vi "getSetup.vi"(7 "Monochromator in":T1={"Type"=enum."PTI", "Wavelength (nm)"=0.0, "Grating, gr/mm"=enum."2400", "Grating mode"=enum."Unknown", "Spectrum mode"={"Spectrum mode?"=FALSE, "Start wavelength (nm)"=0.0, "End wavelength (nm)"=0.0, "Wavelength step (nm)"=0.0, "Wavelength array"=[], "array index"=0}, "PTI"={"Delay before read (ms)"=0, "Mono 1"={"Timeout (ms)"=0, "Resource Name"="", "Baud Rate"=0, "Data Bits"=0, "Parity"=0, "Stop Bits"=0, "Flow Control"=0}, "Mono 2"={"Timeout (ms)"=0, "Resource Name"="", "Baud Rate"=0, "Data Bits"=0, "Parity"=0, "Stop Bits"=0, "Flow Control"=0}, "Two PTI Monochromators?"=FALSE}, "Oriel (custom)"={"reference"=refnum}, "Force wavelength confirmation (PTI)?"=FALSE} {"PTI"."Mono 2"."Flow Control" items=["1.0"=10, "1.5"=15, "2.0"=20]; "PTI"."Mono 2"."Stop Bits" items=["None", "Odd", "Even", "Mark", "Space"]; "PTI"."Mono 2"."Parity" items=["None", "Odd", "Even", "Mark", "Space"]; "PTI"."Mono 1"."Flow Control" items=["1.0"=10, "1.5"=15, "2.0"=20]; "PTI"."Mono 1"."Stop Bits" items=["None", "Odd", "Even", "Mark", "Space"]; "PTI"."Mono 1"."Parity" items=["None", "Odd", "Even", "Mark", "Space"]}, 8 "error in (no error)":errorcluster, 11 "Enable wavelength input? (T)":bool) -> (0 "error out":errorcluster={"status"=FALSE, "code"=1073676294, "source"="VISA Read in Monochromator.lvlib:ReadWrite.vi->Monochromator.lvlib:move.vi:1990001->Monochromator.lvlib:moveBothMonos.vi->Monochromator.lvlib:Main.vi"}, 5 "Monochromator out":T1 {"PTI"."Mono 2"."Flow Control" items=["1.0"=10, "1.5"=15, "2.0"=20]; "PTI"."Mono 2"."Stop Bits" items=["None", "Odd", "Even", "Mark", "Space"]; "PTI"."Mono 2"."Parity" items=["None", "Odd", "Even", "Mark", "Space"]; "PTI"."Mono 1"."Flow Control" items=["1.0"=10, "1.5"=15, "2.0"=20]; "PTI"."Mono 1"."Stop Bits" items=["None", "Odd", "Even", "Mark", "Space"]; "PTI"."Mono 1"."Parity" items=["None", "Odd", "Even", "Mark", "Space"]})   [LabVIEW 2017, in "Monochromator.lvlib"]
doc: "Gets the current wavelength via either user input (with a PTI mononchromator) or by reading it from the monochromator (Oriel monochromator). \nThe PTI-monochromator-mode user input also allows the user to specify the current grating mode (IR/visible). In IR mode, the wavelength entered by the user is multiplied by two to get the current wavelength."
uses:
  Monochromator.lvlib
  Controls/Params.ctl
  Controls/Type.ctl
  Controls/GratingValues.ctl
  Controls/Grating.ctl
  PTI/Controls/Params.ctl
  Controls/VISA parameters.ctl
  Custom Oriel drivers/Controls/Params.ctl
  C:/Project Work/icl-optical-software-rewrite/Optical Software Code Simplified/Modules/Monochromator/Cornerstone.dll
  Cornerstone.dll
  PTI/PTI.lvlib
  Custom Oriel drivers/Oriel (custom drivers).lvlib
  Serial comms/Serial comms.lvlib
panel:
  in  "Is IR":bool caption="Grating"
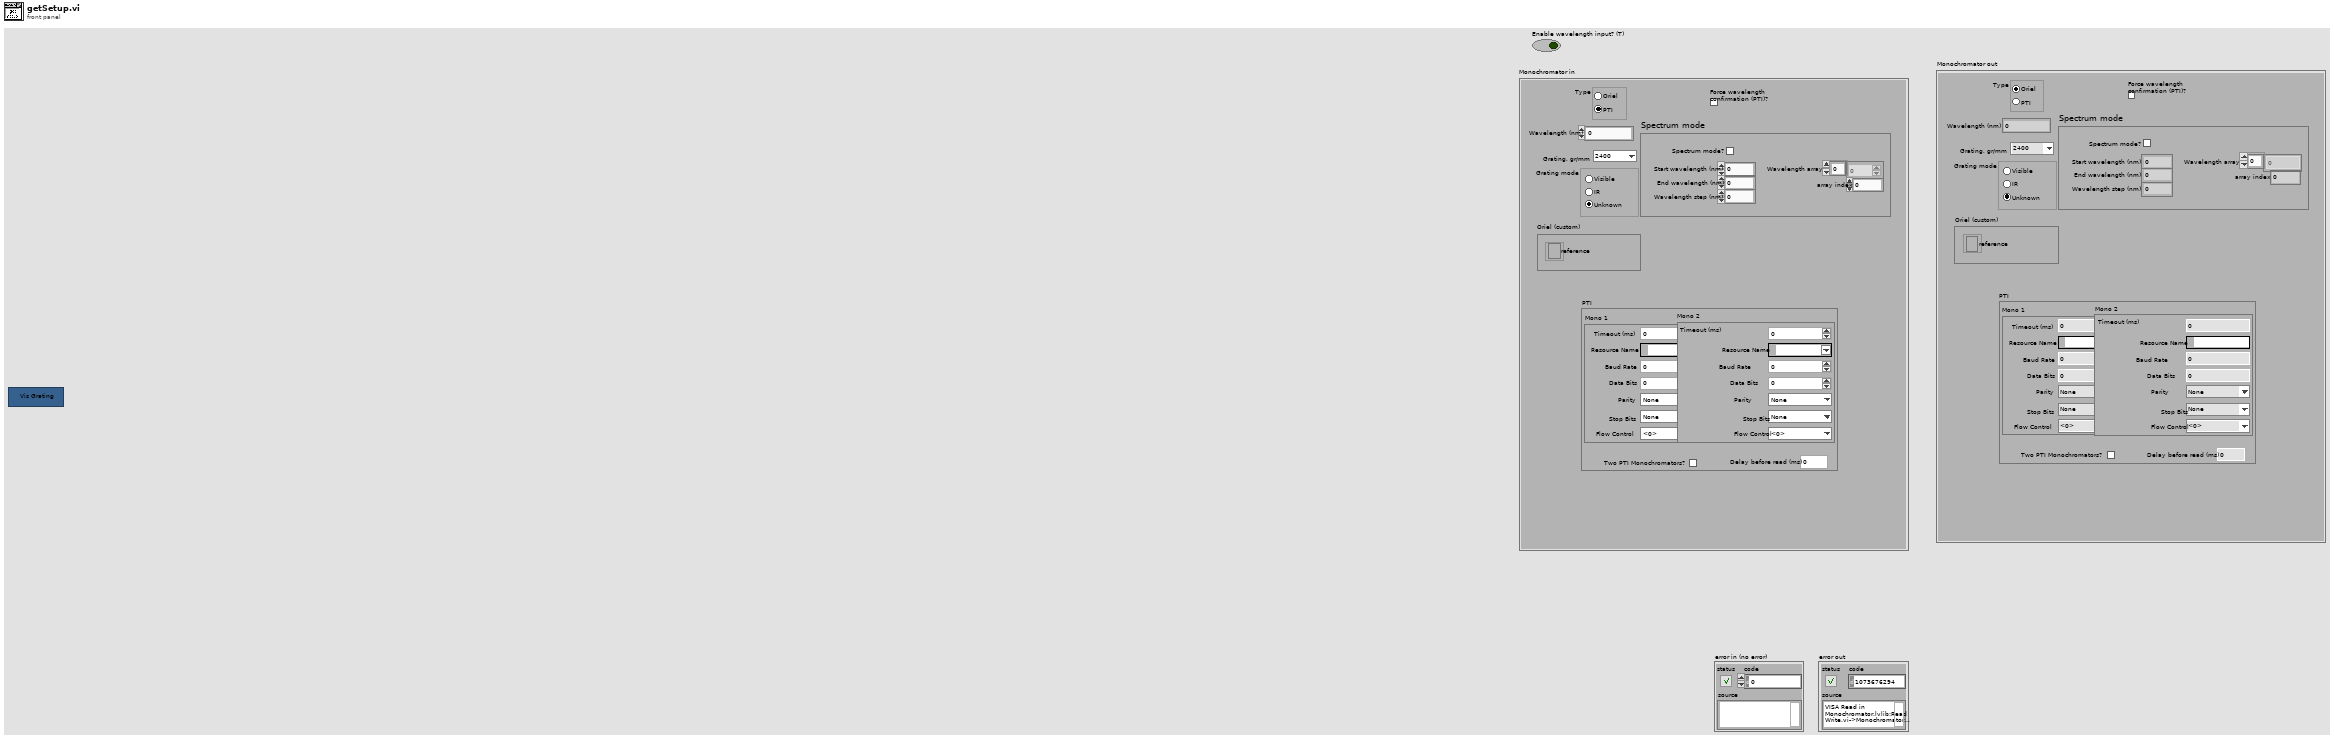
[diagram p1: front panel]
types:
  T1 = typedef "Monochromator.lvlib/Params.ctl" = cluster{"Type":T2, "Wavelength (nm)":dbl, "Grating, gr/mm":T3, "Grating mode":T4, "Spectrum mode":cluster{"Spectrum mode?":bool, "Start wavelength (nm)":dbl, "End wavelength (nm)":dbl, "Wavelength step (nm)":dbl, "Wavelength array":dbl[], "array index":u32}, "PTI":T5, "Oriel (custom)":T7, "Force wavelength confirmation (PTI)?":bool}
  T2 = typedef "Monochromator.lvlib/Type.ctl" = enum32{"Oriel", "PTI"}
  T3 = typedef "Monochromator.lvlib/GratingValues.ctl" = enum16{"2400", "1800", "1200", "600", "300", "150"}
  T4 = typedef "Monochromator.lvlib/Grating.ctl" = enum32{"Unknown", "Visible", "IR"}
  T5 = typedef "Monochromator.lvlib/PTI.lvlib/Params.ctl" = cluster{"Delay before read (ms)":u32, "Mono 1":T6, "Mono 2":T6, "Two PTI Monochromators?":bool}
  T6 = typedef "Serial comms.lvlib/VISA parameters.ctl" = cluster{"Timeout (ms)":u32, "Resource Name":refnum<visa-resource-name>, "Baud Rate":u32, "Data Bits":u16, "Parity":u16, "Stop Bits":u16, "Flow Control":u16}
  T7 = typedef "Monochromator.lvlib/Oriel (custom drivers).lvlib/Params.ctl" = cluster{"reference":refnum<k24>}
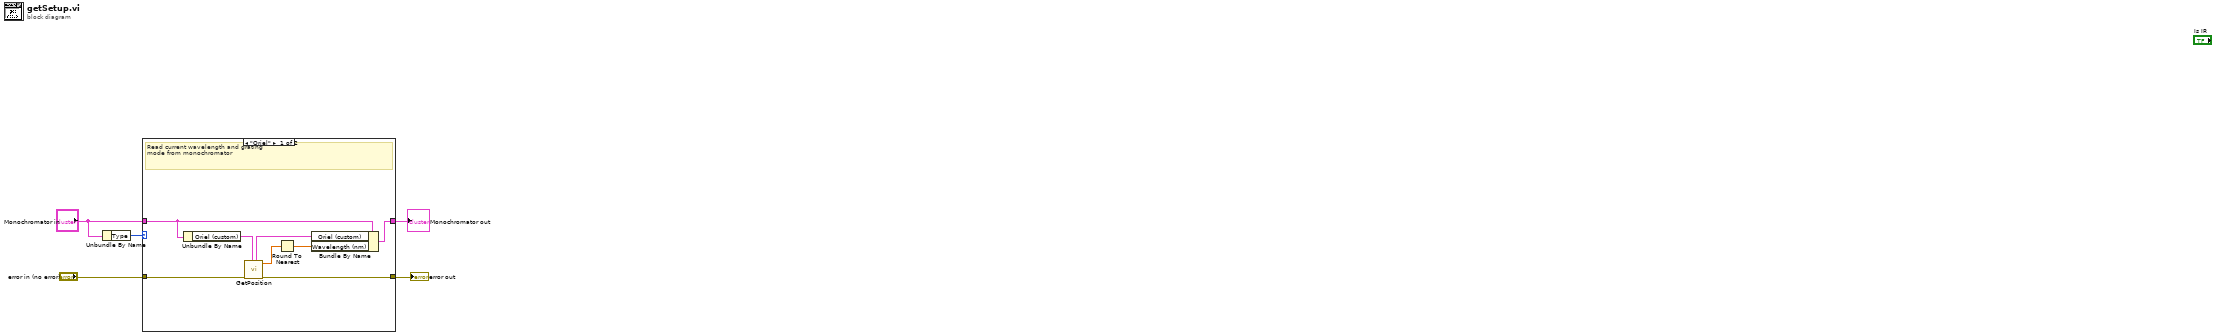
[diagram p0: block diagram]
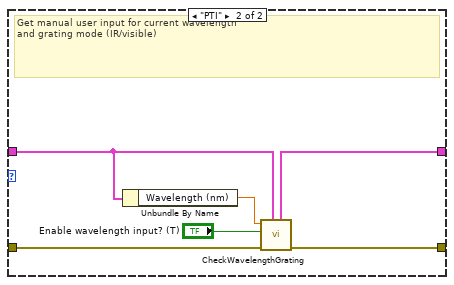
[diagram p2: hidden frame]
diagram:
  n1 = Unbundle By Name("Monochromator in") -> ("Type"=w5:T2)
  n2 = case shown="\"Oriel\"" w5 {
    tunnel: [w10 w18] -> w3
    tunnel: "error in (no error)" -> [w11 w19]
    tunnel: "Monochromator in" -> [w13 w15]
    tunnel: [w12 w16] -> w1
    frame "Oriel" {
      # "Read current wavelength and grating \nmode from monochromator"
      n3 = Unbundle By Name(w13) -> ("Oriel (custom)"=w9:T7)
      n4 = call "GetPosition.vi"("Oriel (custom drivers) in"=w9, "error in (no error)"=w11) -> ("error out"=w10:errorcluster, "Wavelength"=w7:dbl, "Oriel (custom drivers) out"=w8:T7)  [unwired: 7 in]
      n5 = Round To Nearest(number=w7) -> (nearest integer value=w6:dbl)
      n6 = Bundle By Name(cluster=w13, "Oriel (custom)"=w8, "Wavelength (nm)"=w6) -> (w12:T1)
    }
    frame "PTI" {
      # "Get manual user input for current wavelength\nand grating mode (IR/visible)"
      n7 = Unbundle By Name(w15) -> ("Wavelength (nm)"=w14:dbl)
      n8 = call "CheckWavelengthGrating.vi"("Monochromator in"=w15, "error in (no error)"=w19, "Enable wavelength input? (F)"="Enable wavelength input? (T)", "Wavelength (nm)"=w14) -> ("error out"=w18:errorcluster, "Monochromator out"=w16:T1)  [unwired: 6 in]
    }
  }
  "Monochromator out" <- w1
  "error out" <- w3
